vi "Build Existing Panel Map.vi"(11 "Panels":refnum<class "ArrayPanel.lvclass">[](array[class])) -> (3 "Existing Panel Map":T1(c390))   [LabVIEW 2020, in "FlexBlocks.lvlib"]
uses:
  FlexBlocks.lvlib
  <vilib>/IlluminatedG/IG OOPanel/OOPanel/ArrayPanel/ArrayPanel.lvclass
  Value Editor Base/Value Editor Base.lvclass
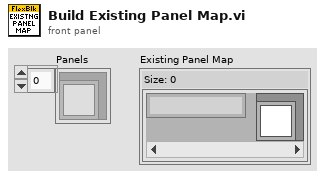
[diagram p1: front panel]
types:
  T1 = map{string, refnum<class "Value Editor Base.lvclass">}
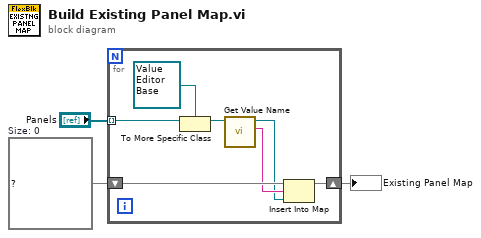
[diagram p0: block diagram]
diagram:
  w2 = T1 {}  # Size: 0
  n1 = for {
    tunnel: "Panels" -> [w10] mode=indexing
    shift-right: [w4] -> w1
    shift-left: w2 -> [w7]
    n2 = To More Specific Class(target class=refnum<class "Value Editor Base.lvclass"> refnum ("FlexBlocks.lvlib:Value Editor Base.lvclass"), reference=w10) -> (specific class reference=w8:refnum<class "Value Editor Base.lvclass">)  [unwired: 1 in, 1 out]
    n3 = call "Get Value Name.vi"("Value Editor Base in"=w8) -> ("Value Name"=w6:string, "Value Editor Base out"=w5:refnum<class "Value Editor Base.lvclass">)  [unwired: 8 in, 1 out]
    n4 = Insert Into Map(map in=w7, key=w6, value=w5) -> (map out=w4:T1)  [unwired: 2 out]
  }
  "Existing Panel Map" <- w1
